vi "CPP-5168-FIDandPressure-Jan2013.vi"() -> (5 "Plug in titles":string[](array[string]), 7 "Plug in values":string[](array[string]))   [LabVIEW 2012]
uses:
  Globals/Meas_global.vi
  <vilib>/measure/mascope.llb/Transition Measurements 1 chan.vi
  <vilib>/measure/NI_MAPro.lvlib
panel:
  out "SourceOffIndex 2":i32
  out "SampleLength 2":i32
  out "SampleLength":i32
  out "ValveShutAt":dbl format="%.2f"
  out "SourceOffIndex":i32
  out "Zeroes?":bool
  out "Zeroes":dbl[](array[numeric])
  out "Data":dbl[][](array[numeric]) caption="ZeroedCompensatedCalibratedData" format="%#_3g"
  out "ChannelNames":string[](array[string])
  # "Use ONLY for combined FID and pressure runs- NOT Pressure-velocity"
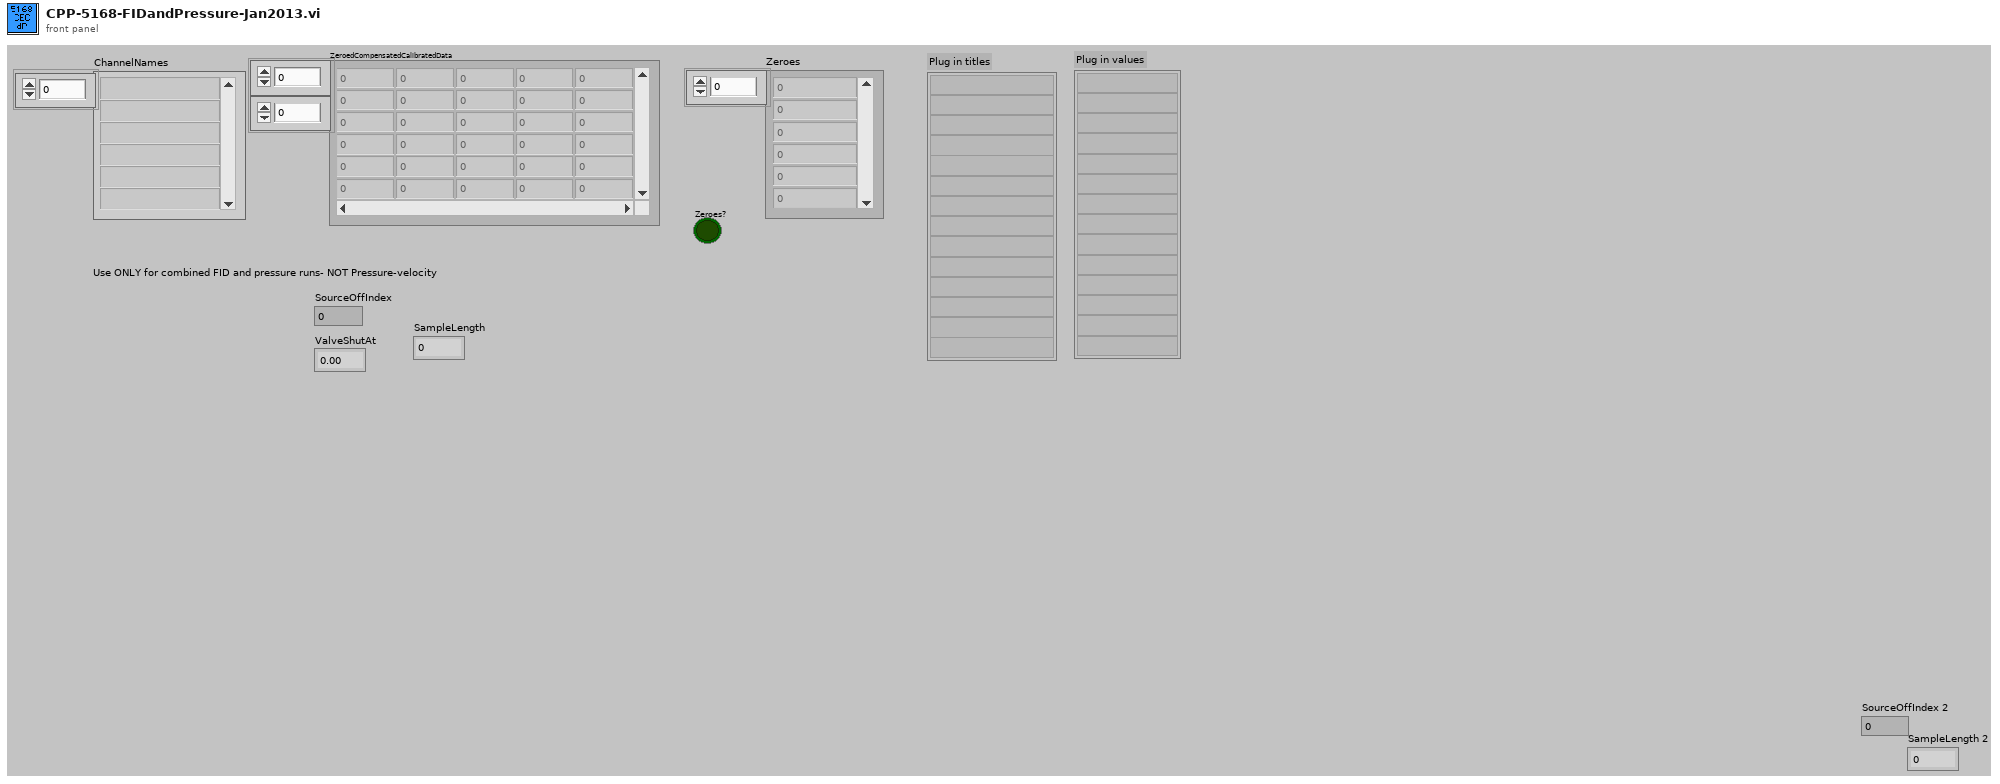
[diagram p1: front panel]
types:
  T1 = typedef "Analysis_info_cluster.ctl" = cluster{"Colour":u32, "Inst type":T2, "Inst name":string, "Symbol":string, "Code name":string, "Extra Info":string, "Inst Array":T3, "Extra Titles":string[], "Extra Values":string[], "U":dbl, "u^2":dbl, "u^3":dbl, "u^4":dbl, "Skew_u":dbl, "Kurt_u":dbl, "Sd Error in Mean":dbl, "% u'/U":dbl, "X":dbl, "Y":dbl, "Z":dbl, "Timescale integral to 25%":dbl, "Sd Error in Variance":dbl, "Calib File":path, "Calib Constants":dbl[], "Output Position":bool, "Full Stats":bool, "Av Sampling Rate":dbl, "Av No of Samples":dbl, "Total Meas Time (s)":dbl, "ADAM Ch Name":string}
  T2 = typedef "Inst_type.ctl" = enum16{"Propeller anemometer", "Raw voltage", "Pressure Transducer", "Pitot-static tube", "Preston tube", "Hot wire", "Cross wire 1", "Cross wire 2", "Generic Linear", "Generic Polynomial", "Generic BackPoly", "Fast FID", "Thermocouple", "Cold wire", "Pulsed Wire", "LDA Vel", "LDA Tran time", "LDA Arr time"}
  T3 = typedef "Instrument_Array.ctl" = enum16{"PWA", "LDA", "Analogue"}
  T4 = typedef "Time_Trace_Cluster.ctl" = cluster{"Weighting":dbl[], "Time (s)":dbl[], "Voltage":dbl[], "Eng Values":dbl[]}
  T5 = cluster{"start time":dbl, "end time":dbl, "ref levels":cluster{"high ref level":dbl, "mid ref level":dbl, "low ref level":dbl, "ref units":u16}}
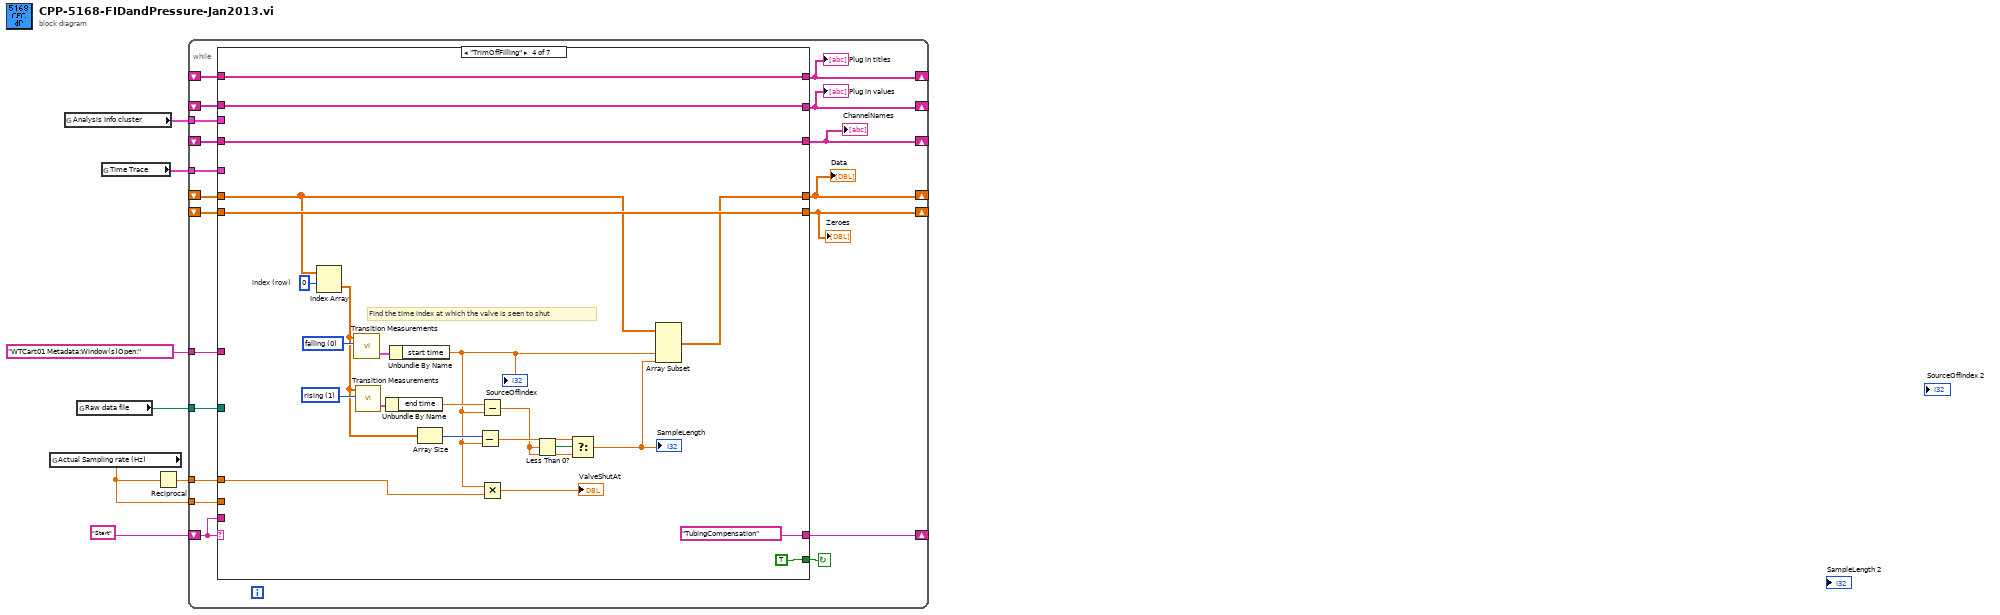
[diagram p0: block diagram]
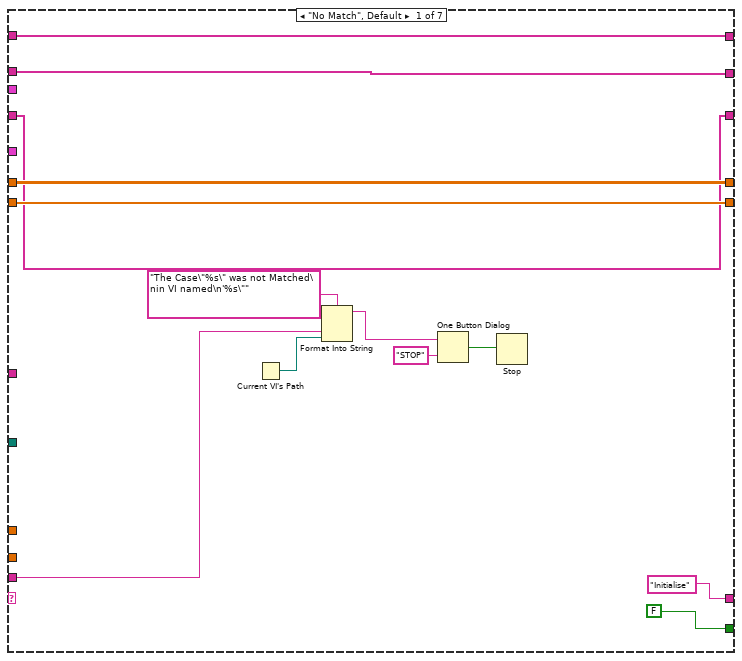
[diagram p2: hidden frame]
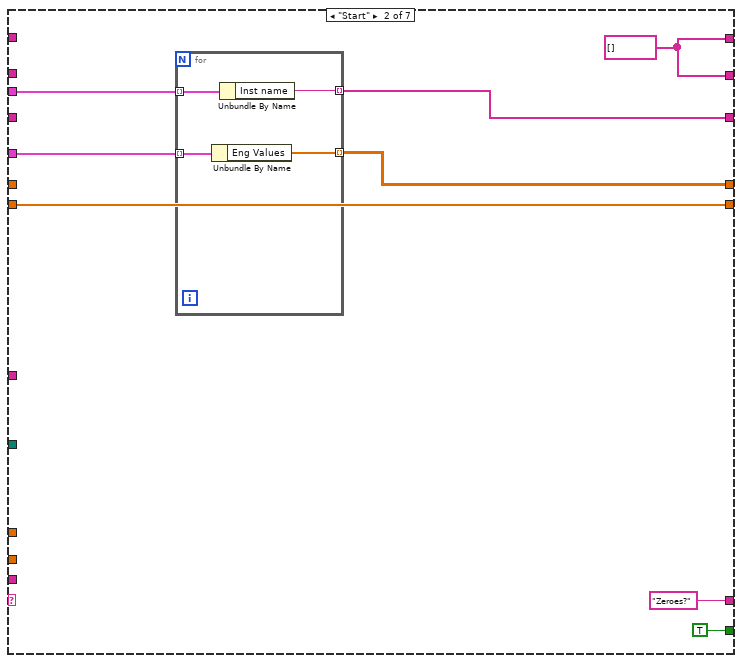
[diagram p3: hidden frame]
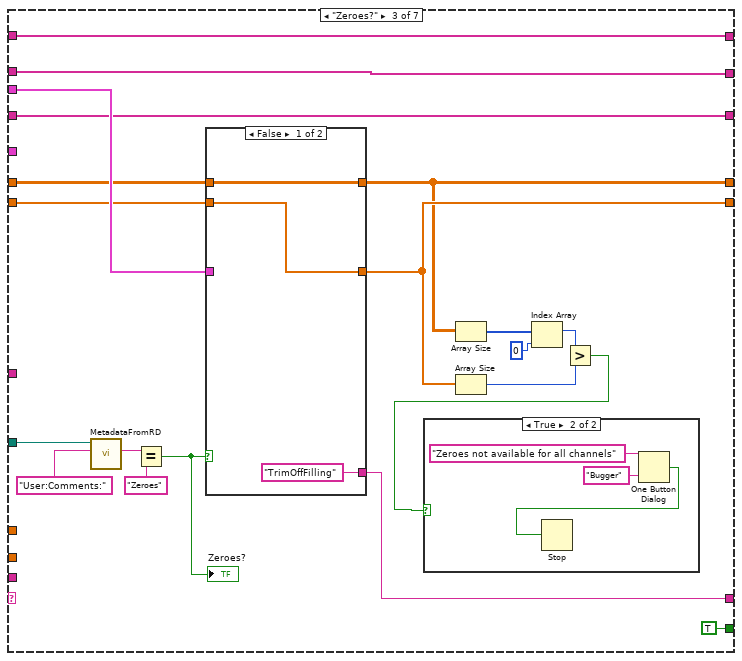
[diagram p4: hidden frame]
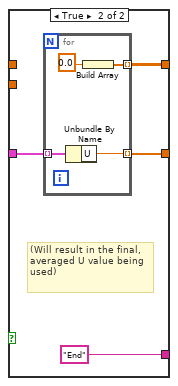
[diagram p6: hidden frame]
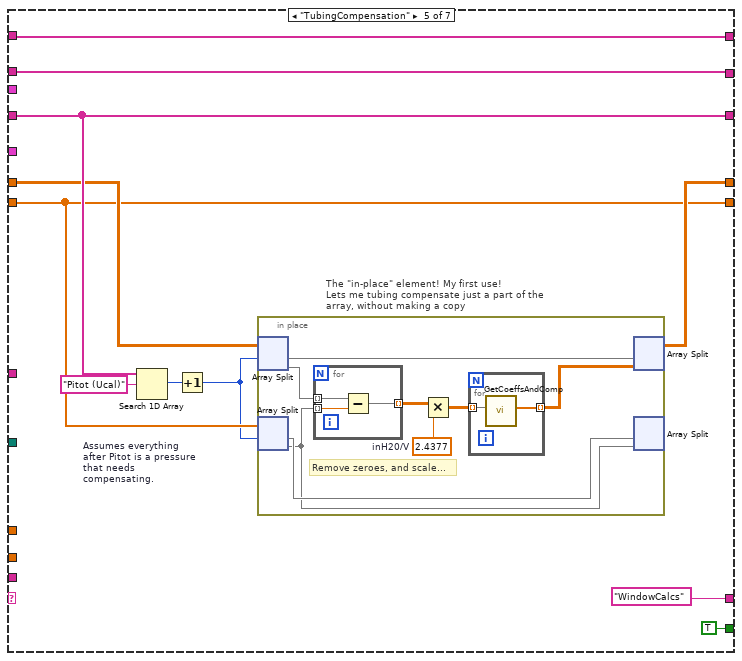
[diagram p7: hidden frame]
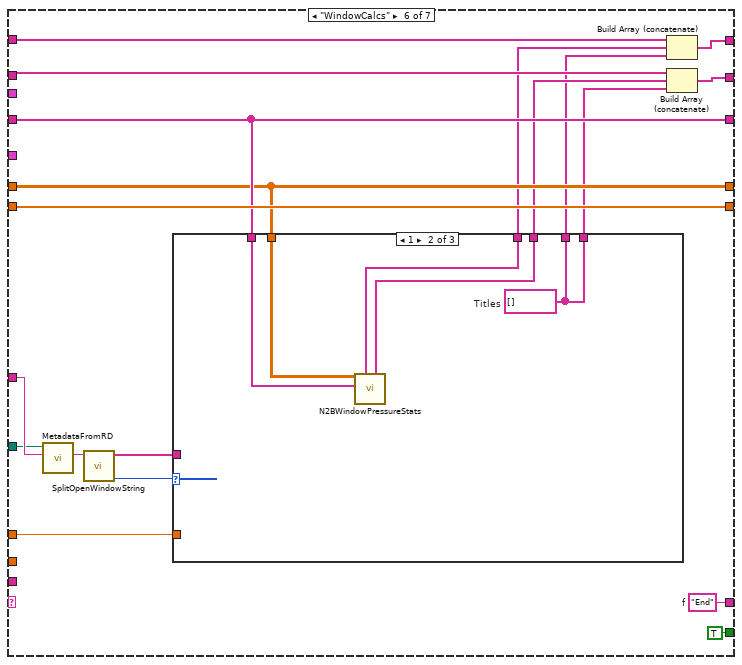
[diagram p8: hidden frame]
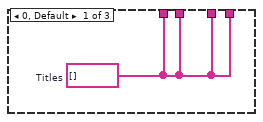
[diagram p9: hidden frame]
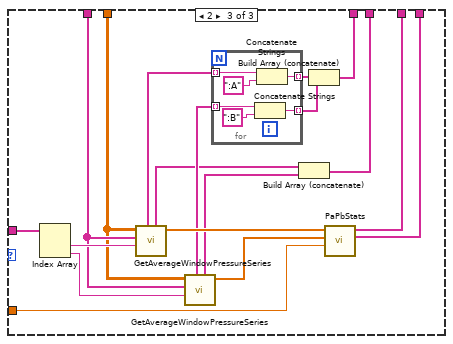
[diagram p10: hidden frame]
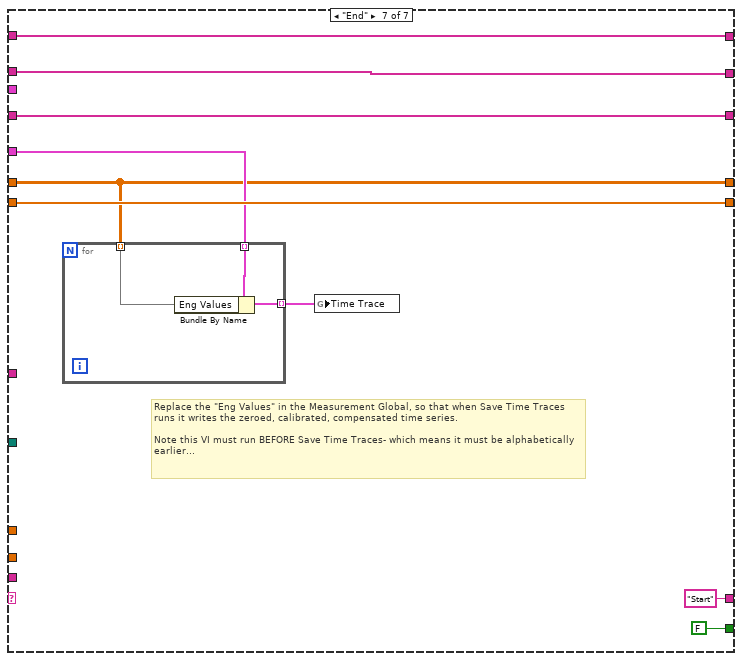
[diagram p11: hidden frame]
diagram:
  n1 = global read "Meas_global.vi" "Actual Sampling rate (Hz)"() -> (w6:dbl)
  n2 = global read "Meas_global.vi" "Analysis Info cluster"() -> (w3:T1[])
  n3 = global read "Meas_global.vi" "Raw data file"() -> (w4:path)
  n4 = global read "Meas_global.vi" "Time Trace"() -> (w2:T4[])
  n5 = Reciprocal(x=w6) -> (1/x=w5:dbl)
  n6 = while {
    shift-left: "Start" -> [w24]
    shift-right: [w25] -> _
    tunnel: w6 -> [w23]
    tunnel: w5 -> [w22]
    tunnel: w4 -> [w19]
    shift-right: [w13] -> _
    shift-left: _ -> [w18]
    shift-right: [w14] -> _
    shift-left: _ -> [w17]
    shift-right: [w16] -> _
    shift-left: _ -> [w15]
    shift-right: [w12] -> _
    shift-left: _ -> [w21]
    tunnel: w3 -> [w11]
    tunnel: w2 -> [w10]
    shift-right: [w9] -> _
    shift-left: _ -> [w20]
    tunnel: "WTCart01 Metadata:Window(s)Open:" -> [w8]
    stop <- w26 continue-if-true
    n7 = case shown="\"TrimOffFilling\"" w24 {
      tunnel: [FALSE TRUE ("Processing last block?") TRUE ("Processing last block?") TRUE TRUE ("Processing last block?") TRUE FALSE ("Processing last block?")] -> w26
      tunnel: ["Initialise" "Zeroes?" w63 "TubingCompensation" ("f") "WindowCalcs" ("f") w147 "Start" ("f")] -> w25
      tunnel: w24 -> [w34 _ _ _ _ _ _]
      tunnel: w23 -> [_ _ _ _ _ _ _]
      tunnel: w22 -> [_ _ _ w94 _ w142 _]
      tunnel: w21 -> [w28 _ w52 w91 w111 w143 w183]
      tunnel: w20 -> [w27 _ w54 w105 w115 w144 w182]
      tunnel: w19 -> [_ _ w71 _ _ w133 _]
      tunnel: w18 -> [w31 _ w69 w108 w113 w151 w188]
      tunnel: [w31 w45 w69 w108 w113 w141 w188] -> w13
      tunnel: [w30 w45 w68 w107 w112 w140 w187] -> w14
      tunnel: w17 -> [w30 _ w68 w107 w112 w139 w187]
      tunnel: [w29 w44 w62 w106 w110 w150 w186] -> w16
      tunnel: w15 -> [w29 w44 w55 w106 w110 w150 w186]
      tunnel: [w28 w42 w53 w90 w114 w143 w183] -> w12
      tunnel: w11 -> [_ w41 w56 _ _ _ _]
      tunnel: w10 -> [_ w43 _ _ _ _ w185]
      tunnel: [w27 w40 w54 w105 w115 w144 w182] -> w9
      tunnel: w8 -> [_ _ _ _ _ w138 _]
      frame "No Match", Default {
        n8 = Current VI's Path() -> (path=w33:path)
        n9 = Format Into String(format string="The Case\"%s\" was not Matched\nin VI named\n'%s\"" ("Format String"), w34, w33) -> (resulting string=w37:string)  [unwired: 2 in, 1 out]
        n10 = One Button Dialog(message=w37, button name ("OK")="STOP") -> (true=w35:bool)
        n11 = Stop(stop? (T)=w35) -> ()
      }
      frame "Start" {
        w45 = string[] []
        n12 = for {
          tunnel: [w50] -> w42 mode=indexing
          tunnel: w43 -> [w51] mode=indexing
          tunnel: w41 -> [w49] mode=indexing
          tunnel: [w48] -> w40 mode=indexing
          n13 = Unbundle By Name(w51) -> ("Eng Values"=w50:dbl[])
          n14 = Unbundle By Name(w49) -> ("Inst name"=w48:string)
        }
      }
      frame "Zeroes?" {
        n15 = call "MetadataFromRD.vi"("ChannelName"="User:Comments:", "Raw data file"=w71) -> ("ValueString"=w66:string)  [unwired: 8 in, 1 out]
        n16 = Equal?(x=w66, y="Zeroes") -> (x = y?=w64:bool)
        "Zeroes?" <- w64
        n17 = case shown="False" w64 {
          tunnel: ["TrimOffFilling" ("f") "End" ("f")] -> w63
          tunnel: [w76 w79] -> w62
          tunnel: w56 -> [_ w80]
          tunnel: w55 -> [w76 _]
          tunnel: [w75 w78] -> w53
          tunnel: w52 -> [w75 _]
          frame False {
          }
          frame True {
            # "(Will result in the final, averaged U value being used)"
            n18 = for {
              tunnel: w80 -> [w85] mode=indexing
              tunnel: [w84] -> w79 mode=indexing
              tunnel: [w82] -> w78 mode=indexing
              n19 = Unbundle By Name(w85) -> ("U"=w84:dbl)
              n20 = Build Array(0.0) -> (w82:dbl[])
            }
          }
        }
        n21 = Array Size(array=w53) -> (size(s)=w61:i32[])
        n22 = Array Size(array=w62) -> (size(s)=w60:i32)
        n23 = Index Array(array=w61, index=0) -> (element=w59:i32)
        n24 = Greater?(x=w59, y=w60) -> (0:w57:bool)
        n25 = case shown="True" w57 {
          frame False {
          }
          frame True {
            n26 = One Button Dialog(message="Zeroes not available for all channels", button name ("OK")="Bugger") -> (true=w72:bool)
            n27 = Stop(stop? (T)=w72) -> ()
          }
        }
      }
      frame "TrimOffFilling" {
        w93 = 0  # index (row)
        w99 = u16 0 items=["falling", "rising"] ("polarity (rising)")
        w98 = u16 1 items=["falling", "rising"] ("polarity (rising)")
        # "Find the time index at which the valve is seen to shut"
        n28 = Index Array(array=w91, index (row)=w93) -> (element=w92:dbl[])  [unwired: 1 in]
        n29 = call-poly <vilib>:"Transition Measurements.vi"("polarity (rising)"=w99, "signal in"=w92) -> ("measurement info"=w95:T5)  [unwired: 4 in, 5 out]
        n30 = call-poly <vilib>:"Transition Measurements.vi"("polarity (rising)"=w98, "signal in"=w92) -> ("measurement info"=w97:T5)  [unwired: 4 in, 5 out]
        n31 = Unbundle By Name(w97) -> ("end time"=w100:dbl)
        n32 = Unbundle By Name(w95) -> ("start time"=w87:dbl)
        "SourceOffIndex" <- w87
        n33 = Array Size(array=w92) -> (size(s)=w103:i32)
        n34 = Subtract(x=w103, y=w87) -> (x-y=w104:dbl)
        n35 = Subtract(x=w100, y=w87) -> (x-y=w102:dbl)
        n36 = Multiply(x=w87, y=w94) -> (x*y=→"ValveShutAt":dbl)
        n37 = Less Than 0?(x=w102) -> (x < 0?=w101:bool)
        n38 = Select(t=w104, s=w101, f=w102) -> (s? t:f=w86:dbl)
        "SampleLength" <- w86
        n39 = Array Subset(array=w91, index (col)=w87, length (col)=w86) -> (w90:dbl[][])  [unwired: 2 in]
      }
      frame "TubingCompensation" {
        n40 = Search 1D Array "Assumes everything after Pitot is a pressure that needs compensating."(1D array=w115, element="Pitot (Ucal)") -> (index of element=w116:i32)  [unwired: 1 in]
        n41 = Increment(x=w116) -> (x+1=w109:i32)
        n42 = in-place "The \"in-place\" element! My first use!\nLets me tubing compensate just a part of the array, without making a copy" {
          w124 = 2.4377  # inH20/V
          # "Remove zeroes, and scale..."
          n43 = in-place-split #1(w111, w109) -> (w127:dbl[][], w123:dbl[][])
          n44 = in-place-split #2(w110, w109) -> (w121:dbl[], w120:dbl[])
          n45 = for {
            tunnel: [w130] -> w122 mode=indexing
            tunnel: w123 -> [w129] mode=indexing
            tunnel: w120 -> [w128] mode=indexing
            n46 = Subtract(x=w129, y=w128) -> (x-y=w130:dbl[])
          }
          n47 = Multiply(x=w122, y=w124) -> (x*y=w125:dbl[][])
          n48 = for {
            tunnel: w125 -> [w132] mode=indexing
            tunnel: [w131] -> w126 mode=indexing
            n49 = call "GetCoeffsAndComp.vi"("mutedData"=w132) -> ("boostedData"=w131:dbl[])  [unwired: 10 in]
          }
          n50 = in-place-split #1(w127, w126) -> (w114:dbl[][])  [unwired: 1 out]
          n51 = in-place-split #2(w121, w120) -> ()  [unwired: 2 out]
        }
      }
      frame "WindowCalcs" {
        w147 = "End"  # f
        n52 = call "MetadataFromRD.vi"("ChannelName"=w138, "Raw data file"=w133) -> ("ValueString"=w149:string)  [unwired: 8 in, 1 out]
        n53 = call "SplitOpenWindowString.vi"("WindowOpenString"=w149) -> ("nWindows"=w146:i32, "OpenWindows"=w145:string[])  [unwired: 9 in]
        n54 = case shown="1" w146 {
          tunnel: w145 -> [_ _ w175]
          tunnel: w144 -> [_ w155 w172]
          tunnel: w143 -> [_ w156 w171]
          tunnel: w142 -> [_ _ w168]
          tunnel: [w152 w157 w167] -> w134
          tunnel: [w152 w157 w166] -> w136
          tunnel: [w152 w154 w159] -> w135
          tunnel: [w152 w153 w158] -> w137
          frame 0, Default {
            w152 = string[] []  # Titles
          }
          frame 1 {
            w157 = string[] []  # Titles
            n55 = call "N2BWindowPressureStats.vi"("ChannelNames"=w155, "ZeroedScaledCompensatedData"=w156) -> ("Values"=w153:string[], "Titles"=w154:string[])  [unwired: 8 in]
          }
          frame 2 {
            n56 = Index Array(array=w175) -> (element #1=w174:string, element #2=w173:string)  [unwired: 2 in]
            n57 = call "GetAverageWindowPressureSeries.vi"("WindowOpenString"=w174, "ChannelNames"=w172, "ZeroedScaledCompensatedData"=w171) -> ("AveragePressureSeries"=w170:dbl[], "Values"=w161:string[], "Titles"=w165:string[])  [unwired: 6 in]
            n58 = call "GetAverageWindowPressureSeries.vi"("WindowOpenString"=w173, "ChannelNames"=w172, "ZeroedScaledCompensatedData"=w171) -> ("AveragePressureSeries"=w169:dbl[], "Values"=w160:string[], "Titles"=w164:string[])  [unwired: 6 in]
            n59 = for {
              tunnel: w165 -> [w181] mode=indexing
              tunnel: w164 -> [w178] mode=indexing
              tunnel: [w177] -> w163 mode=indexing
              tunnel: [w176] -> w162 mode=indexing
              n60 = Concatenate Strings(w178, ":B" ("string")) -> (w176:string)
              n61 = Concatenate Strings(w181, ":A" ("string")) -> (w177:string)
            }
            n62 = Build Array (concatenate)(w161, w160) -> (w158:string[])
            n63 = Build Array (concatenate)(w163, w162) -> (w159:string[])
            n64 = call "PaPbStats.vi"("dT"=w168, "TimeseriesB"=w169, "TimeseriesA"=w170) -> ("Values"=w166:string[], "Titles"=w167:string[])  [unwired: 7 in]
          }
        }
        n65 = Build Array (concatenate)(w151, w135, w134) -> (w141:string[])
        n66 = Build Array (concatenate)(w139, w137, w136) -> (w140:string[])
      }
      frame "End" {
        # "Replace the \"Eng Values\" in the Measurement Global, so that when Save Time Traces runs it writes the zeroed, calibrated, compensated time series.\n\nNote this VI must run BEFORE Save Time Traces- which means it must be alphabetically earlier..."
        n67 = for {
          tunnel: w185 -> [w193] mode=indexing
          tunnel: [w192] -> w184 mode=indexing
          tunnel: w183 -> [w191] mode=indexing
          n68 = Bundle By Name(cluster=w193, "Eng Values"=w191) -> (w192:T4)
        }
        n69 = global write "Meas_global.vi" "Time Trace"(w184) -> ()
      }
    }
    "Plug in values" <- w14
    "Plug in titles" <- w13
    "Data" <- w12
    "Zeroes" <- w16
    "ChannelNames" <- w9
  }
